vi "TranslatorBooster Check if Variable Name.vi"(4 "String":string) -> (1 "Is Type?":bool, 2 "ref or ptr":string)   [LabVIEW 2014, in "Complex Numbers.lvlib"]
uses:
  <vilib>/Aledyne-TSXperts/Arduino Compatible Compiler for LabVIEW/addons/Complex Numbers/Complex Numbers.lvlib
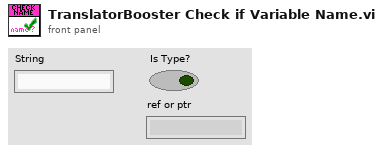
[diagram p1: front panel]
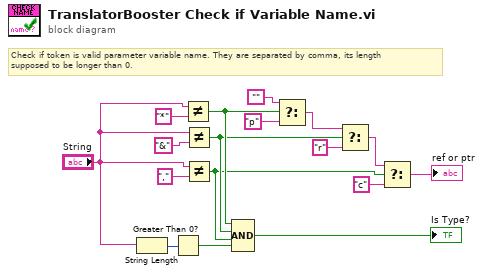
[diagram p0: block diagram]
diagram:
  # "Check if token is valid parameter variable name. They are separated by comma, its length\nsupposed to be longer than 0."
  n1 = String Length(string="String") -> (length=w17:i32)
  n2 = Greater Than 0?(x=w17) -> (x > 0?=w15:bool)
  n3 = Not Equal?(x="String", y="*") -> (x != y?=w10:bool)
  n4 = Not Equal?(x="String", y="&") -> (x != y?=w7:bool)
  n5 = Not Equal?(x="String", y=",") -> (x != y?=w2:bool)
  n6 = Compound Arithmetic op=AND(w10, w7, w2, w15) -> (→"Is Type?":bool)
  n7 = Select(t="", s=w10, f="p") -> (s? t:f=w5:string)
  n8 = Select(t=w5, s=w7, f="r") -> (s? t:f=w1:string)
  n9 = Select(t=w1, s=w2, f="c") -> (s? t:f=→"ref or ptr":string)
